vi "Check Matlab Mode Error.vi"(8 "error in":errorcluster, 10 "custom error string (empty)":string) -> (0 "error out":errorcluster)   [LabVIEW 2013, in "GOLPI library.lvlib"]
doc: "This will check error generated by the Matlab script node. If detected, it will be converted to undestandable form unlike the original which does no sense. \nThe VI has also input for custom error string. It has priority over the input error line so if the string is no empty, it will override input error."
uses:
  GOLPI library.lvlib
  Type Definitions/Custom Error Codes Enum Type Def.vi
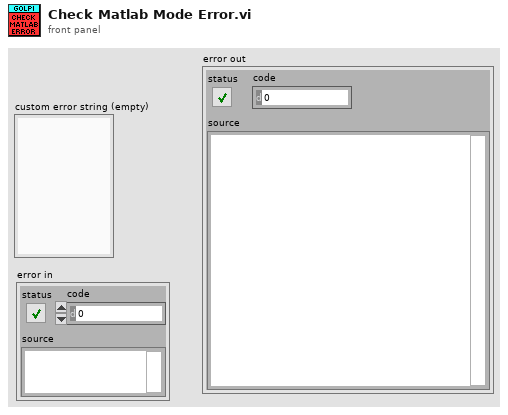
[diagram p1: front panel]
types:
  T1 = typedef "GOLPI library.lvlib/Custom Error Codes Enum Type Def.vi" = enum16{"no error", "00 working directory PAR1 missing", "01 octave binary PAR1 missing", "02 octave report error PAR1", "03 empty output last cmd PAR1", "04 missing temporary file PAR1", "05 pwd PAR 1 not exist", "06 oct package not installed", "10 var PAR1 not string, vect", "11 var PAR1 not num, scal, ~compl", "12 var PAR1 not num, scal, compl", "13 var PAR1 not num, vect, ~compl", "14 var PAR1 not num, vect, compl", "15 var PAR1 not num, mat, ~compl", "16 var PAR1 not num, mat, ~compl", "30 read timeout", "60 bitstream transport failed", "61 bitstream decode error PAR1", "62 bitstream cannot be set", "70 struct transfer not possible", "80 struct: cluster elem. PAR1 not implem.", "81 struct: structure field PAR1 not implem.", "82 struct: size mismatch of PAR1", "83 struct: type mismatch of PAR1", "98 internal error", "99 not finished", "90 Not supported in Matlab mode", "91 Matlab variable transfer error", "92 Matlab Script Error"}
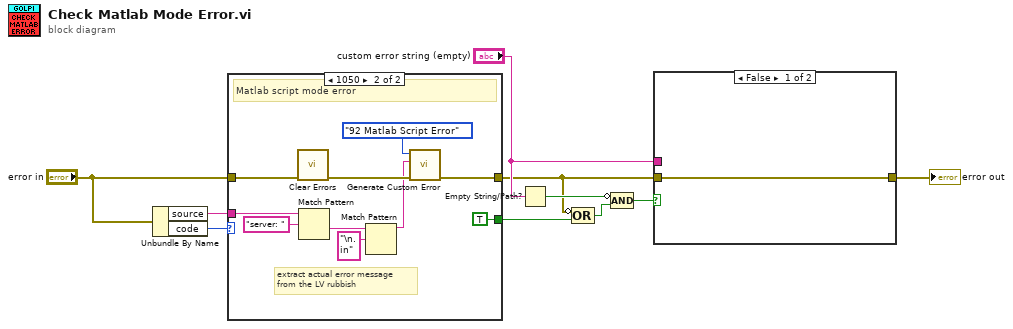
[diagram p0: block diagram]
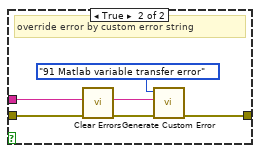
[diagram p2: hidden frame]
diagram:
  n1 = Unbundle By Name("error in") -> ("source"=w10:string, "code"=w9:i32)
  n2 = case shown="1050" w9 {
    tunnel: w10 -> [_ w21]
    tunnel: "error in" -> [w11 w17]
    tunnel: [w11 w13] -> w4
    tunnel: [_ TRUE] -> w3
    frame Default {
      # "general error - do not modify"
    }
    frame 1050 {
      # "extract actual error message\nfrom the LV rubbish"
      # "Matlab script mode error"
      n3 = call <vilib>:"Clear Errors.vi"("error in (no error)"=w17) -> ("error out"=w16:errorcluster)  [unwired: 6 in]
      n4 = Match Pattern(string=w21, regular expression="server: ") -> (after substring=w19:string)  [unwired: 1 in, 3 out]
      n5 = Match Pattern(string=w19, regular expression="\n. in") -> (before substring=w15:string)  [unwired: 1 in, 3 out]
      n6 = call "Generate Custom Error.vi"("error in"=w16, "PAR1"=w15, "GOLPI error"=Custom_Error_Codes_Enum_Type_Def.vi."92 Matlab Script Error") -> ("error out"=w13:errorcluster)  [unwired: 8 in]
    }
  }
  n7 = Empty String/Path?(string/path="custom error string (empty)") -> (empty?=w5:bool)
  n8 = Compound Arithmetic op=OR(invert w4, w3) -> (w2:bool)
  n9 = Compound Arithmetic op=AND(invert w5, w2) -> (w1:bool)
  n10 = case shown="False" w1 {
    tunnel: w4 -> [w22 w25]
    tunnel: "custom error string (empty)" -> [_ w26]
    tunnel: [w22 w23] -> w7
    frame False {
    }
    frame True {
      # "override error by custom error string"
      n11 = call <vilib>:"Clear Errors.vi"("error in (no error)"=w25) -> ("error out"=w24:errorcluster)  [unwired: 6 in]
      n12 = call "Generate Custom Error.vi"("error in"=w24, "PAR1"=w26, "GOLPI error"=Custom_Error_Codes_Enum_Type_Def.vi."91 Matlab variable transfer error") -> ("error out"=w23:errorcluster)  [unwired: 8 in]
    }
  }
  "error out" <- w7
